vi "Definition Cluster.vi"(11 "Timestamp in":refnum<class "Timestamp.lvclass">) -> (2 "Definition":variant, 3 "Timestamp out":refnum<class "Timestamp.lvclass">)   [LabVIEW 2020, in "Conditum.lvlib" / "Columns.lvlib" / "Timestamp.lvclass"]
uses:
  Timestamp.lvclass
  Timestamp.lvclass/Timestamp.ctl
  Attributes.ctl
  Conditum.lvlib
  Type/Definition.ctl
  Type/Type.lvclass
  Definition.ctl
  Timestamp Definition.ctl
  C:/dev/lv20CE/lv-conditum/Conditum/Columns/Type/Type.lvclass
  C:/dev/lv20CE/lv-conditum/Conditum/Columns/Timestamp/Timestamp.lvclass
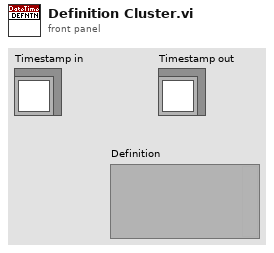
[diagram p1: front panel]
types:
  T1 = typedef "Conditum.lvlib/Columns.lvlib/Timestamp.lvclass/Timestamp Definition.ctl" = cluster{"Type":T2, "Attributes":T3, "Timestamp":T4}
  T2 = typedef "Conditum.lvlib/Columns.lvlib/Type.lvclass/Definition.ctl" = cluster{"Name":string, "Nullable":bool, "Default NULL":bool}
  T3 = typedef "Conditum.lvlib/Attributes.ctl" = cluster{"Primary Key":bool, "Unique":bool, "Foreign Key":bool, "Auto Increment":bool}
  T4 = typedef "Conditum.lvlib/Columns.lvlib/Timestamp.lvclass/Definition.ctl" = cluster{"Default":timestamp}
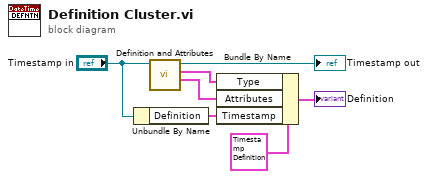
[diagram p0: block diagram]
diagram:
  n1 = Unbundle By Name("Timestamp in") -> ("Definition"=w6:T4)
  n2 = call "Definition and Attributes.vi"("Type in"="Timestamp in") -> ("Attributes"=w4:T3, "Definition"=w5:T2, "Type out"=→"Timestamp out":refnum<class "Timestamp.lvclass">)  [unwired: 8 in]
  n3 = Bundle By Name(cluster=T1 {"Type"={"Name"="", "Nullable"=FALSE, "Default NULL"=FALSE}, "Attributes"={"Primary Key"=FALSE, "Unique"=FALSE, "Foreign Key"=FALSE, "Auto Increment"=FALSE}, "Timestamp"={"Default"=timestamp(0 s since 1904-01-01)}} ("Definition"), "Type"=w5, "Attributes"=w4, "Timestamp"=w6) -> (→"Definition":T1)
